vi "user process.vi"(8 "error in":errorcluster, 11 "Parameters to process":T2) -> (0 "error out":errorcluster, 3 "Results from processing":T1)   [LabVIEW 2017, in "GPIC Core runtime.lvclass"]
uses:
  GPIC Core runtime.lvclass
  parameter user data.ctl
  result user data.ctl
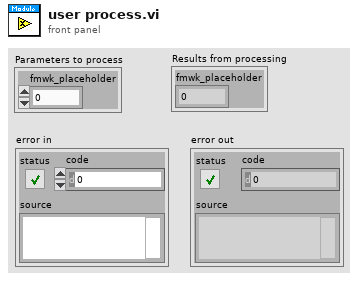
[diagram p1: front panel]
types:
  T1 = typedef "GPIC Core runtime.lvclass/result user data.ctl" = cluster{"fmwk_placeholder":i32}
  T2 = typedef "GPIC Core runtime.lvclass/parameter user data.ctl" = cluster{"fmwk_placeholder":i32}
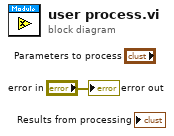
[diagram p0: block diagram]
diagram:
  "error out" <- "error in"
